vi "输入数据解析.vi"(0 "单个参数补充":dbl, 1 "从板号":dbl=1.0, 2 "主板二维码":string="BNET01", 3 "从板二维码":string="BNET01", 5 "主板引用":refnum<vi>, 7 "从板引用":refnum<vi>, 9 "主板选项":string="三级故障阀值", 11 "枚举":enum16{"主板", "从板"}(ring), 12 "快换":bool caption="快换写入") -> (4 "输出数组":dbl[][](array[numeric]), 6 "数组长度":dbl[](array[numeric]), 8 "循环次数":i32, 10 "命令":u32, 14 "名称":string[](array[string]), 15 "命令序号":u32[](array[numeric]))   [LabVIEW 2013] (continued)
                  frame Enabled {
                  }
                }
                n1001 = Build Array(w2456) -> (w2455:i32[])
              }
              frame 5 {
                # "单组电压不均衡"
                n1002 = disable-structure shown="启用" {
                  disable-tunnel: [w2472 w2475] -> w2467
                  disable-tunnel: [w2470 w2475] -> w2465
                  disable-tunnel: w2464 -> [w2469 _]
                  frame Disabled {
                    n1003 = Unbundle By Name(w2469) -> ("单组电压不均衡"=w2468:dbl)
                    n1004 = call "输入分辨率计算-EV05.vi"("1字节?"=FALSE, "数值"=w2468, "偏移量"=0.0, "分辨率"=0.001) -> ("低字节"=w2470:dbl, "高字节1"=w2472:dbl)  [unwired: 1 in, 5 out]
                  }
                  frame Enabled {
                    w2475 = 255 ("高字节1")
                  }
                }
                n1005 = Build Array(w2467, w2465) -> (w2466:i32[])
              }
              frame 6 {
                # "整组电压不均衡"
                n1006 = disable-structure shown="启用" {
                  disable-tunnel: [w2484 w2487] -> w2479
                  disable-tunnel: [w2482 w2487] -> w2477
                  disable-tunnel: w2476 -> [w2481 _]
                  frame Disabled {
                    n1007 = Unbundle By Name(w2481) -> ("整组电压不均衡"=w2480:dbl)
                    n1008 = call "输入分辨率计算-EV05.vi"("1字节?"=FALSE, "数值"=w2480, "偏移量"=0.0, "分辨率"=0.001) -> ("低字节"=w2482:dbl, "高字节1"=w2484:dbl)  [unwired: 1 in, 5 out]
                  }
                  frame Enabled {
                    w2487 = 255 ("高字节1")
                  }
                }
                n1009 = Build Array(w2479, w2477) -> (w2478:i32[])
              }
              frame 7 {
                # "单体电压过高"
                n1010 = disable-structure shown="启用" {
                  disable-tunnel: [w2496 w2499] -> w2491
                  disable-tunnel: [w2494 w2499] -> w2489
                  disable-tunnel: w2488 -> [w2493 _]
                  frame Disabled {
                    n1011 = Unbundle By Name(w2493) -> ("单体电压过高"=w2492:dbl)
                    n1012 = call "输入分辨率计算-EV05.vi"("1字节?"=FALSE, "数值"=w2492, "偏移量"=0.0, "分辨率"=0.001) -> ("低字节"=w2494:dbl, "高字节1"=w2496:dbl)  [unwired: 1 in, 5 out]
                  }
                  frame Enabled {
                    w2499 = 255 ("高字节1")
                  }
                }
                n1013 = Build Array(w2491, w2489) -> (w2490:i32[])
              }
              frame 8 {
                # "单体电压过低"
                n1014 = disable-structure shown="启用" {
                  disable-tunnel: [w2508 w2511] -> w2503
                  disable-tunnel: [w2506 w2511] -> w2501
                  disable-tunnel: w2500 -> [w2505 _]
                  frame Disabled {
                    n1015 = Unbundle By Name(w2505) -> ("单体电压过低"=w2504:dbl)
                    n1016 = call "输入分辨率计算-EV05.vi"("1字节?"=FALSE, "数值"=w2504, "偏移量"=0.0, "分辨率"=0.001) -> ("低字节"=w2506:dbl, "高字节1"=w2508:dbl)  [unwired: 1 in, 5 out]
                  }
                  frame Enabled {
                    w2511 = 255 ("高字节1")
                  }
                }
                n1017 = Build Array(w2503, w2501) -> (w2502:i32[])
              }
              frame 9 {
                # "充电电流过高"
                n1018 = disable-structure shown="启用" {
                  disable-tunnel: [w2520 w2523] -> w2515
                  disable-tunnel: [w2518 w2523] -> w2513
                  disable-tunnel: w2512 -> [w2517 _]
                  frame Disabled {
                    n1019 = Unbundle By Name(w2517) -> ("充电电流过高"=w2516:dbl)
                    n1020 = call "输入分辨率计算-EV05.vi"("1字节?"=FALSE, "数值"=w2516, "偏移量"=-3000.0, "分辨率"=0.1) -> ("低字节"=w2518:dbl, "高字节1"=w2520:dbl)  [unwired: 1 in, 5 out]
                  }
                  frame Enabled {
                    w2523 = 255 ("高字节1")
                  }
                }
                n1021 = Build Array(w2515, w2513) -> (w2514:i32[])
              }
              frame 10 {
                # "放电电流过高"
                n1022 = disable-structure shown="启用" {
                  disable-tunnel: [w2532 w2535] -> w2527
                  disable-tunnel: [w2530 w2535] -> w2525
                  disable-tunnel: w2524 -> [w2529 _]
                  frame Disabled {
                    n1023 = Unbundle By Name(w2529) -> ("放电电流过高"=w2528:dbl)
                    n1024 = call "输入分辨率计算-EV05.vi"("1字节?"=FALSE, "数值"=w2528, "偏移量"=-3000.0, "分辨率"=0.1) -> ("低字节"=w2530:dbl, "高字节1"=w2532:dbl)  [unwired: 1 in, 5 out]
                  }
                  frame Enabled {
                    w2535 = 255 ("高字节1")
                  }
                }
                n1025 = Build Array(w2527, w2525) -> (w2526:i32[])
              }
              frame 11 {
                # "单组温度不均衡"
                n1026 = disable-structure shown="启用" {
                  disable-tunnel: [w2542 255 ("高字节1")] -> w2538
                  disable-tunnel: w2536 -> [w2540 _]
                  frame Disabled {
                    n1027 = Unbundle By Name(w2540) -> ("单组温度不均衡"=w2539:dbl)
                    n1028 = call "输入分辨率计算-EV05.vi"("1字节?"=TRUE, "数值"=w2539, "偏移量"=0.0, "分辨率"=1.0) -> ("高字节1"=w2542:dbl)  [unwired: 1 in, 6 out]
                  }
                  frame Enabled {
                  }
                }
                n1029 = Build Array(w2538) -> (w2537:i32[])
              }
              frame 12 {
                # "SOC过高"
                n1030 = Unbundle By Name(w2550) -> ("SOC过高"=w2549:dbl)
                n1031 = call "输入分辨率计算-EV05.vi"("1字节?"=FALSE, "数值"=w2549, "偏移量"=0.0, "分辨率"=0.1) -> ("低字节"=w2551:dbl, "高字节1"=w2552:dbl)  [unwired: 1 in, 5 out]
                n1032 = call "二进制解析-8.6.vi"("索引"=4, "数值"=w2552) -> ("低位子数组"=w2555:i32[])  [unwired: 3 out]
                n1033 = call "二进制解析-8.6.vi"("索引"=4, "数值"=w2551) -> ("低位子数组"=w2547:i32[], "高位子数组"=w2554:i32[])  [unwired: 2 out]
                n1034 = Insert Into Array(array=w2555, new element=w2554) -> (w2553:i32[])  [unwired: 1 in]
                n1035 = call "数值二进制转十进制-8.6.vi"("子数组"=w2553) -> ("十进制数值"=w2548:i32)  [unwired: 4 out]
                n1036 = disable-structure shown="启用" {
                  disable-tunnel: w2548 -> [w2563 _]
                  disable-tunnel: [w2563 255 ("高字节1")] -> w2546
                  disable-tunnel: [w2562 i32[] [] ("低位子数组 20")] -> _
                  disable-tunnel: w2547 -> [w2562 _]
                  frame Disabled {
                  }
                  frame Enabled {
                  }
                }
                n1037 = Build Array(w2546, w2546) -> (w2559:i32[])
              }
              frame 13 {
                # "SOC过低"
                n1038 = Unbundle By Name(w2572) -> ("SOC过低"=w2571:dbl)
                n1039 = call "输入分辨率计算-EV05.vi"("1字节?"=FALSE, "数值"=w2571, "偏移量"=0.0, "分辨率"=0.1) -> ("低字节"=w2569:dbl, "高字节1"=w2570:dbl)  [unwired: 1 in, 5 out]
                n1040 = call "二进制解析-8.6.vi"("索引"=4, "数值"=w2570) -> ("低位子数组"=w2567:i32[])  [unwired: 3 out]
                n1041 = disable-structure shown="启用" {
                  disable-tunnel: w2569 -> [w2579 _]
                  disable-tunnel: [w2579 255 ("高字节1")] -> w2568
                  disable-tunnel: w2567 -> [w2578 _]
                  disable-tunnel: [_ 255 ("高字节1")] -> w2566
                  frame Disabled {
                    (unwired) i32[] [] ("低位子数组 4")
                  }
                  frame Enabled {
                  }
                }
                n1042 = Build Array(w2566, w2568) -> (w2575:i32[])
              }
              frame 14 {
                # "内阻过大"
                n1043 = disable-structure shown="启用" {
                  disable-tunnel: w2584 -> [w2589 _]
                  disable-tunnel: [w2585 255 ("高字节1")] -> w2582
                  frame Disabled {
                    n1044 = Unbundle By Name(w2589) -> ("内阻过大"=w2588:dbl)
                    n1045 = call "输入分辨率计算-EV05.vi"("1字节?"=TRUE, "数值"=w2588, "分辨率"=0.1) -> ("高字节1"=w2585:dbl)  [unwired: 2 in, 6 out]
                  }
                  frame Enabled {
                  }
                }
                n1046 = Build Array(w2582) -> (w2583:i32[])
              }
              frame 15 {
                # "极柱温度过高"
                n1047 = disable-structure shown="启用" {
                  disable-tunnel: w2593 -> [w2599 _]
                  disable-tunnel: [w2595 255 ("高字节1")] -> w2591
                  frame Disabled {
                    n1048 = Unbundle By Name(w2599) -> ("极柱温度过高"=w2598:dbl)
                    n1049 = call "输入分辨率计算-EV05.vi"("1字节?"=TRUE, "数值"=w2598, "偏移量"=-40.0, "分辨率"=1.0) -> ("高字节1"=w2595:dbl)  [unwired: 1 in, 6 out]
                  }
                  frame Enabled {
                  }
                }
                n1050 = Build Array(w2591) -> (w2592:i32[])
              }
              frame 16 {
                # "SOH过低"
                n1051 = disable-structure shown="启用" {
                  disable-tunnel: [w2616 w2624] -> w2603
                  disable-tunnel: w2602 -> [w2613 _]
                  disable-tunnel: [w2605 w2624] -> w2601
                  frame Disabled {
                    n1052 = Unbundle By Name(w2613) -> ("SOH过低"=w2612:dbl)
                    n1053 = call "输入分辨率计算-EV05.vi"("1字节?"=FALSE, "数值"=w2612, "偏移量"=0.0, "分辨率"=0.1) -> ("低字节"=w2614:dbl, "高字节1"=w2615:dbl)  [unwired: 1 in, 5 out]
                    n1054 = call "二进制解析-8.6.vi"("索引"=4, "数值"=w2615) -> ("低位子数组"=w2618:i32[])  [unwired: 3 out]
                    n1055 = call "二进制解析-8.6.vi"("索引"=4, "数值"=w2614) -> ("低位子数组"=w2607:i32[], "高位子数组"=w2617:i32[])  [unwired: 2 out]
                    n1056 = call "二进制解析-8.6.vi"("索引"=4, "数值"=0) -> ("低位子数组"=w2608:i32[])  [unwired: 3 out]
                    n1057 = Insert Into Array(array=w2618, new element=w2617) -> (w2611:i32[])  [unwired: 1 in]
                    n1058 = Insert Into Array(array=w2607, new element=w2608) -> (w2606:i32[])  [unwired: 1 in]
                    n1059 = call "数值二进制转十进制-8.6.vi"("子数组"=w2611) -> ("十进制数值"=w2616:i32)  [unwired: 4 out]
                    n1060 = call "数值二进制转十进制-8.6.vi"("子数组"=w2606) -> ("十进制数值"=w2605:i32)  [unwired: 4 out]
                  }
                  frame Enabled {
                    w2624 = 255 ("高字节1")
                  }
                }
                n1061 = Build Array(w2603, w2601) -> (w2604:i32[])
              }
            }
            n1062 = Insert Into Array(array=w2408, new element=w2409) -> (w2407:dbl[])  [unwired: 1 in]
          }
          n1063 = Build Array(w2404) -> (w2403:dbl[][])
          n1064 = Build Array("三级故障阀值") -> (w2394:string[])
        }
        frame "温度过高(2)" {
          n1065 = Unbundle By Name(w2630) -> ("一级故障 2"=w2631:refnum<vi>)
          n1066 = property class="Clust (严格)"(reference=w2631) -> ("Value"=w2629:T4)  [unwired: 1 in, 2 out]
          n1067 = for {
            N: 17 -> [_]
            tunnel: w2629 -> [w2641]
            shift-right: [w2638] -> w2635
            shift-left: dbl[] [] -> [w2639]
            i -> [w2642]
            n1068 = case shown="13" w2642 {
              tunnel: w2641 -> [w2643 w2654 w2665 w2675 w2685 w2695 w2707 w2719 w2731 w2743 w2755 w2767 w2781 w2803 w2815 w2824 w2833]
              tunnel: [w2644 w2655 w2666 w2676 w2686 w2697 w2709 w2721 w2733 w2745 w2757 w2768 w2790 w2806 w2814 w2823 w2835] -> w2640
              frame 0, Default {
                # "总电压过高"
                n1069 = disable-structure shown="启用" {
                  disable-tunnel: [w2650 w2653] -> w2646
                  disable-tunnel: [w2649 w2653] -> w2645
                  disable-tunnel: w2643 -> [w2648 _]
                  frame Disabled {
                    n1070 = Unbundle By Name(w2648) -> ("总电压过高"=w2647:dbl)
                    n1071 = call "输入分辨率计算-EV05.vi"("1字节?"=FALSE, "数值"=w2647, "分辨率"=0.1) -> ("低字节"=w2650:dbl, "高字节1"=w2649:dbl)  [unwired: 2 in, 5 out]
                  }
                  frame Enabled {
                    w2653 = 255 ("高字节1")
                  }
                }
                n1072 = Build Array(w2645, w2646) -> (w2644:i32[])
              }
              frame 1 {
                # "总电压过低"
                n1073 = disable-structure shown="启用" {
                  disable-tunnel: [w2661 w2664] -> w2657
                  disable-tunnel: [w2660 w2664] -> w2656
                  disable-tunnel: w2654 -> [w2659 _]
                  frame Disabled {
                    n1074 = Unbundle By Name(w2659) -> ("总电压过低"=w2658:dbl)
                    n1075 = call "输入分辨率计算-EV05.vi"("1字节?"=FALSE, "数值"=w2658, "分辨率"=0.1) -> ("低字节"=w2661:dbl, "高字节1"=w2660:dbl)  [unwired: 2 in, 5 out]
                  }
                  frame Enabled {
                    w2664 = 255 ("高字节1")
                  }
                }
                n1076 = Build Array(w2656, w2657) -> (w2655:i32[])
              }
              frame 2 {
                # "温度过高"
                n1077 = disable-structure shown="启用" {
                  disable-tunnel: [w2671 255 ("高字节1")] -> w2667
                  disable-tunnel: w2665 -> [w2669 _]
                  frame Enabled {
                    n1078 = Unbundle By Name(w2669) -> ("温度过高"=w2668:dbl)
                    n1079 = call "输入分辨率计算-EV05.vi"("1字节?"=TRUE, "数值"=w2668, "偏移量"=-40.0, "分辨率"=1.0) -> ("高字节1"=w2671:dbl)  [unwired: 1 in, 6 out]
                  }
                  frame Disabled {
                  }
                }
                n1080 = Build Array(w2667) -> (w2666:dbl[])
              }
              frame 3 {
                # "温度过低"
                n1081 = disable-structure shown="启用" {
                  disable-tunnel: [w2681 255 ("高字节1")] -> w2677
                  disable-tunnel: w2675 -> [w2679 _]
                  frame Disabled {
                    n1082 = Unbundle By Name(w2679) -> ("温度过低"=w2678:dbl)
                    n1083 = call "输入分辨率计算-EV05.vi"("1字节?"=TRUE, "数值"=w2678, "偏移量"=-40.0, "分辨率"=1.0) -> ("高字节1"=w2681:dbl)  [unwired: 1 in, 6 out]
                  }
                  frame Enabled {
                  }
                }
                n1084 = Build Array(w2677) -> (w2676:i32[])
              }
              frame 4 {
                # "整组温度不均衡"
                n1085 = disable-structure shown="启用" {
                  disable-tunnel: [w2691 255 ("高字节1")] -> w2687
                  disable-tunnel: w2685 -> [w2689 _]
                  frame Disabled {
                    n1086 = Unbundle By Name(w2689) -> ("整组温度不均衡"=w2688:dbl)
                    n1087 = call "输入分辨率计算-EV05.vi"("1字节?"=TRUE, "数值"=w2688, "偏移量"=0.0, "分辨率"=1.0) -> ("高字节1"=w2691:dbl)  [unwired: 1 in, 6 out]
                  }
                  frame Enabled {
                  }
                }
                n1088 = Build Array(w2687) -> (w2686:i32[])
              }
              frame 5 {
                # "单组电压不均衡"
                n1089 = disable-structure shown="启用" {
                  disable-tunnel: [w2703 w2706] -> w2698
                  disable-tunnel: [w2701 w2706] -> w2696
                  disable-tunnel: w2695 -> [w2700 _]
                  frame Disabled {
                    n1090 = Unbundle By Name(w2700) -> ("单组电压不均衡"=w2699:dbl)
                    n1091 = call "输入分辨率计算-EV05.vi"("1字节?"=FALSE, "数值"=w2699, "偏移量"=0.0, "分辨率"=0.001) -> ("低字节"=w2701:dbl, "高字节1"=w2703:dbl)  [unwired: 1 in, 5 out]
                  }
                  frame Enabled {
                    w2706 = 255 ("高字节1")
                  }
                }
                n1092 = Build Array(w2698, w2696) -> (w2697:i32[])
              }
              frame 6 {
                # "整组电压不均衡"
                n1093 = disable-structure shown="启用" {
                  disable-tunnel: [w2715 w2718] -> w2710
                  disable-tunnel: [w2713 w2718] -> w2708
                  disable-tunnel: w2707 -> [w2712 _]
                  frame Disabled {
                    n1094 = Unbundle By Name(w2712) -> ("整组电压不均衡"=w2711:dbl)
                    n1095 = call "输入分辨率计算-EV05.vi"("1字节?"=FALSE, "数值"=w2711, "偏移量"=0.0, "分辨率"=0.001) -> ("低字节"=w2713:dbl, "高字节1"=w2715:dbl)  [unwired: 1 in, 5 out]
                  }
                  frame Enabled {
                    w2718 = 255 ("高字节1")
                  }
                }
                n1096 = Build Array(w2710, w2708) -> (w2709:i32[])
              }
              frame 7 {
                # "单体电压过高"
                n1097 = disable-structure shown="启用" {
                  disable-tunnel: [w2727 w2730] -> w2722
                  disable-tunnel: [w2725 w2730] -> w2720
                  disable-tunnel: w2719 -> [w2724 _]
                  frame Disabled {
                    n1098 = Unbundle By Name(w2724) -> ("单体电压过高"=w2723:dbl)
                    n1099 = call "输入分辨率计算-EV05.vi"("1字节?"=FALSE, "数值"=w2723, "偏移量"=0.0, "分辨率"=0.001) -> ("低字节"=w2725:dbl, "高字节1"=w2727:dbl)  [unwired: 1 in, 5 out]
                  }
                  frame Enabled {
                    w2730 = 255 ("高字节1")
                  }
                }
                n1100 = Build Array(w2722, w2720) -> (w2721:i32[])
              }
              frame 8 {
                # "单体电压过低"
                n1101 = disable-structure shown="启用" {
                  disable-tunnel: [w2739 w2742] -> w2734
                  disable-tunnel: [w2737 w2742] -> w2732
                  disable-tunnel: w2731 -> [w2736 _]
                  frame Disabled {
                    n1102 = Unbundle By Name(w2736) -> ("单体电压过低"=w2735:dbl)
                    n1103 = call "输入分辨率计算-EV05.vi"("1字节?"=FALSE, "数值"=w2735, "偏移量"=0.0, "分辨率"=0.001) -> ("低字节"=w2737:dbl, "高字节1"=w2739:dbl)  [unwired: 1 in, 5 out]
                  }
                  frame Enabled {
                    w2742 = 255 ("高字节1")
                  }
                }
                n1104 = Build Array(w2734, w2732) -> (w2733:i32[])
              }
              frame 9 {
                # "充电电流过高"
                n1105 = disable-structure shown="启用" {
                  disable-tunnel: [w2751 w2754] -> w2746
                  disable-tunnel: [w2749 w2754] -> w2744
                  disable-tunnel: w2743 -> [w2748 _]
                  frame Disabled {
                    n1106 = Unbundle By Name(w2748) -> ("充电电流过高"=w2747:dbl)
                    n1107 = call "输入分辨率计算-EV05.vi"("1字节?"=FALSE, "数值"=w2747, "偏移量"=-3000.0, "分辨率"=0.1) -> ("低字节"=w2749:dbl, "高字节1"=w2751:dbl)  [unwired: 1 in, 5 out]
                  }
                  frame Enabled {
                    w2754 = 255 ("高字节1")
                  }
                }
                n1108 = Build Array(w2746, w2744) -> (w2745:i32[])
              }
              frame 10 {
                # "放电电流过高"
                n1109 = disable-structure shown="启用" {
                  disable-tunnel: [w2763 w2766] -> w2758
                  disable-tunnel: [w2761 w2766] -> w2756
                  disable-tunnel: w2755 -> [w2760 _]
                  frame Disabled {
                    n1110 = Unbundle By Name(w2760) -> ("放电电流过高"=w2759:dbl)
                    n1111 = call "输入分辨率计算-EV05.vi"("1字节?"=FALSE, "数值"=w2759, "偏移量"=-3000.0, "分辨率"=0.1) -> ("低字节"=w2761:dbl, "高字节1"=w2763:dbl)  [unwired: 1 in, 5 out]
                  }
                  frame Enabled {
                    w2766 = 255 ("高字节1")
                  }
                }
                n1112 = Build Array(w2758, w2756) -> (w2757:i32[])
              }
              frame 11 {
                # "单组温度不均衡"
                n1113 = disable-structure shown="启用" {
                  disable-tunnel: [w2773 255 ("高字节1")] -> w2769
                  disable-tunnel: w2767 -> [w2771 _]
                  frame Disabled {
                    n1114 = Unbundle By Name(w2771) -> ("单组温度不均衡"=w2770:dbl)
                    n1115 = call "输入分辨率计算-EV05.vi"("1字节?"=TRUE, "数值"=w2770, "偏移量"=0.0, "分辨率"=1.0) -> ("高字节1"=w2773:dbl)  [unwired: 1 in, 6 out]
                  }
                  frame Enabled {
                  }
                }
                n1116 = Build Array(w2769) -> (w2768:i32[])
              }
              frame 12 {
                # "SOC过高"
                n1117 = Unbundle By Name(w2781) -> ("SOC过高"=w2780:dbl)
                n1118 = call "输入分辨率计算-EV05.vi"("1字节?"=FALSE, "数值"=w2780, "偏移量"=0.0, "分辨率"=0.1) -> ("低字节"=w2782:dbl, "高字节1"=w2783:dbl)  [unwired: 1 in, 5 out]
                n1119 = call "二进制解析-8.6.vi"("索引"=4, "数值"=w2783) -> ("低位子数组"=w2786:i32[])  [unwired: 3 out]
                n1120 = call "二进制解析-8.6.vi"("索引"=4, "数值"=w2782) -> ("低位子数组"=w2778:i32[], "高位子数组"=w2785:i32[])  [unwired: 2 out]
                n1121 = Insert Into Array(array=w2786, new element=w2785) -> (w2784:i32[])  [unwired: 1 in]
                n1122 = call "数值二进制转十进制-8.6.vi"("子数组"=w2784) -> ("十进制数值"=w2779:i32)  [unwired: 4 out]
                n1123 = disable-structure shown="启用" {
                  disable-tunnel: w2779 -> [w2794 _]
                  disable-tunnel: [w2794 255 ("高字节1")] -> w2777
                  disable-tunnel: [w2793 i32[] [] ("低位子数组 20")] -> _
                  disable-tunnel: w2778 -> [w2793 _]
                  frame Disabled {
                  }
                  frame Enabled {
                  }
                }
                n1124 = Build Array(w2777, w2777) -> (w2790:i32[])
              }
              frame 13 {
                # "SOC过低"
                n1125 = Unbundle By Name(w2803) -> ("SOC过低"=w2802:dbl)
                n1126 = call "输入分辨率计算-EV05.vi"("1字节?"=FALSE, "数值"=w2802, "偏移量"=0.0, "分辨率"=0.1) -> ("低字节"=w2800:dbl, "高字节1"=w2801:dbl)  [unwired: 1 in, 5 out]
                n1127 = call "二进制解析-8.6.vi"("索引"=4, "数值"=w2801) -> ("低位子数组"=w2798:i32[])  [unwired: 3 out]
                n1128 = disable-structure shown="启用" {
                  disable-tunnel: w2800 -> [w2810 _]
                  disable-tunnel: [w2810 255 ("高字节1")] -> w2799
                  disable-tunnel: w2798 -> [w2809 _]
                  disable-tunnel: [_ 255 ("高字节1")] -> w2797
                  frame Disabled {
                    (unwired) i32[] [] ("低位子数组 4")
                  }
                  frame Enabled {
                  }
                }
                n1129 = Build Array(w2797, w2799) -> (w2806:i32[])
              }
              frame 14 {
                # "内阻过大"
                n1130 = disable-structure shown="启用" {
                  disable-tunnel: w2815 -> [w2820 _]
                  disable-tunnel: [w2816 255 ("高字节1")] -> w2813
                  frame Disabled {
                    n1131 = Unbundle By Name(w2820) -> ("内阻过大"=w2819:dbl)
                    n1132 = call "输入分辨率计算-EV05.vi"("1字节?"=TRUE, "数值"=w2819, "分辨率"=0.1) -> ("高字节1"=w2816:dbl)  [unwired: 2 in, 6 out]
                  }
                  frame Enabled {
                  }
                }
                n1133 = Build Array(w2813) -> (w2814:i32[])
              }
              frame 15 {
                # "极柱温度过高"
                n1134 = disable-structure shown="启用" {
                  disable-tunnel: w2824 -> [w2830 _]
                  disable-tunnel: [w2826 255 ("高字节1")] -> w2822
                  frame Disabled {
                    n1135 = Unbundle By Name(w2830) -> ("极柱温度过高"=w2829:dbl)
                    n1136 = call "输入分辨率计算-EV05.vi"("1字节?"=TRUE, "数值"=w2829, "偏移量"=-40.0, "分辨率"=1.0) -> ("高字节1"=w2826:dbl)  [unwired: 1 in, 6 out]
                  }
                  frame Enabled {
                  }
                }
                n1137 = Build Array(w2822) -> (w2823:i32[])
              }
              frame 16 {
                # "SOH过低"
                n1138 = disable-structure shown="启用" {
                  disable-tunnel: [w2847 w2855] -> w2834
                  disable-tunnel: w2833 -> [w2844 _]
                  disable-tunnel: [w2836 w2855] -> w2832
                  frame Disabled {
                    n1139 = Unbundle By Name(w2844) -> ("SOH过低"=w2843:dbl)
                    n1140 = call "输入分辨率计算-EV05.vi"("1字节?"=FALSE, "数值"=w2843, "偏移量"=0.0, "分辨率"=0.1) -> ("低字节"=w2845:dbl, "高字节1"=w2846:dbl)  [unwired: 1 in, 5 out]
                    n1141 = call "二进制解析-8.6.vi"("索引"=4, "数值"=w2846) -> ("低位子数组"=w2849:i32[])  [unwired: 3 out]
                    n1142 = call "二进制解析-8.6.vi"("索引"=4, "数值"=w2845) -> ("低位子数组"=w2838:i32[], "高位子数组"=w2848:i32[])  [unwired: 2 out]
                    n1143 = call "二进制解析-8.6.vi"("索引"=4, "数值"=0) -> ("低位子数组"=w2839:i32[])  [unwired: 3 out]
                    n1144 = Insert Into Array(array=w2849, new element=w2848) -> (w2842:i32[])  [unwired: 1 in]
                    n1145 = Insert Into Array(array=w2838, new element=w2839) -> (w2837:i32[])  [unwired: 1 in]
                    n1146 = call "数值二进制转十进制-8.6.vi"("子数组"=w2842) -> ("十进制数值"=w2847:i32)  [unwired: 4 out]
                    n1147 = call "数值二进制转十进制-8.6.vi"("子数组"=w2837) -> ("十进制数值"=w2836:i32)  [unwired: 4 out]
                  }
                  frame Enabled {
                    w2855 = 255 ("高字节1")
                  }
                }
                n1148 = Build Array(w2834, w2832) -> (w2835:i32[])
              }
            }
            n1149 = Insert Into Array(array=w2639, new element=w2640) -> (w2638:dbl[])  [unwired: 1 in]
          }
          n1150 = Build Array(w2635) -> (w2634:dbl[][])
          n1151 = Build Array("二级故障阀值") -> (w2625:string[])
        }
        frame "温度过高(3)" {
          n1152 = Unbundle By Name(w2861) -> ("一级故障 3"=w2862:refnum<vi>)
          n1153 = property class="Clust (严格)"(reference=w2862) -> ("Value"=w2860:T4)  [unwired: 1 in, 2 out]
          n1154 = for {
            N: 17 -> [_]
            tunnel: w2860 -> [w2872]
            shift-right: [w2869] -> w2866
            shift-left: dbl[] [] -> [w2870]
            i -> [w2873]
            n1155 = case shown="13" w2873 {
              tunnel: w2872 -> [w2874 w2885 w2896 w2906 w2916 w2926 w2938 w2950 w2962 w2974 w2986 w2998 w3012 w3034 w3046 w3055 w3064]
              tunnel: [w2875 w2886 w2897 w2907 w2917 w2928 w2940 w2952 w2964 w2976 w2988 w2999 w3021 w3037 w3045 w3054 w3066] -> w2871
              frame 0, Default {
                # "总电压过高"
                n1156 = disable-structure shown="启用" {
                  disable-tunnel: [w2881 w2884] -> w2877
                  disable-tunnel: [w2880 w2884] -> w2876
                  disable-tunnel: w2874 -> [w2879 _]
                  frame Disabled {
                    n1157 = Unbundle By Name(w2879) -> ("总电压过高"=w2878:dbl)
                    n1158 = call "输入分辨率计算-EV05.vi"("1字节?"=FALSE, "数值"=w2878, "分辨率"=0.1) -> ("低字节"=w2881:dbl, "高字节1"=w2880:dbl)  [unwired: 2 in, 5 out]
                  }
                  frame Enabled {
                    w2884 = 255 ("高字节1")
                  }
                }
                n1159 = Build Array(w2876, w2877) -> (w2875:i32[])
              }
              frame 1 {
                # "总电压过低"
                n1160 = disable-structure shown="启用" {
                  disable-tunnel: [w2892 w2895] -> w2888
                  disable-tunnel: [w2891 w2895] -> w2887
                  disable-tunnel: w2885 -> [w2890 _]
                  frame Disabled {
                    n1161 = Unbundle By Name(w2890) -> ("总电压过低"=w2889:dbl)
                    n1162 = call "输入分辨率计算-EV05.vi"("1字节?"=FALSE, "数值"=w2889, "分辨率"=0.1) -> ("低字节"=w2892:dbl, "高字节1"=w2891:dbl)  [unwired: 2 in, 5 out]
                  }
                  frame Enabled {
                    w2895 = 255 ("高字节1")
                  }
                }
                n1163 = Build Array(w2887, w2888) -> (w2886:i32[])
              }
              frame 2 {
                # "温度过高"
                n1164 = disable-structure shown="启用" {
                  disable-tunnel: [w2902 255 ("高字节1")] -> w2898
                  disable-tunnel: w2896 -> [w2900 _]
                  frame Enabled {
                    n1165 = Unbundle By Name(w2900) -> ("温度过高"=w2899:dbl)
                    n1166 = call "输入分辨率计算-EV05.vi"("1字节?"=TRUE, "数值"=w2899, "偏移量"=-40.0, "分辨率"=1.0) -> ("高字节1"=w2902:dbl)  [unwired: 1 in, 6 out]
                  }
                  frame Disabled {
                  }
                }
                n1167 = Build Array(w2898) -> (w2897:dbl[])
              }
              frame 3 {
                # "温度过低"
                n1168 = disable-structure shown="启用" {
                  disable-tunnel: [w2912 255 ("高字节1")] -> w2908
                  disable-tunnel: w2906 -> [w2910 _]
                  frame Disabled {
                    n1169 = Unbundle By Name(w2910) -> ("温度过低"=w2909:dbl)
                    n1170 = call "输入分辨率计算-EV05.vi"("1字节?"=TRUE, "数值"=w2909, "偏移量"=-40.0, "分辨率"=1.0) -> ("高字节1"=w2912:dbl)  [unwired: 1 in, 6 out]
                  }
                  frame Enabled {
                  }
                }
                n1171 = Build Array(w2908) -> (w2907:i32[])
              }
              frame 4 {
                # "整组温度不均衡"
                n1172 = disable-structure shown="启用" {
                  disable-tunnel: [w2922 255 ("高字节1")] -> w2918
                  disable-tunnel: w2916 -> [w2920 _]
                  frame Disabled {
                    n1173 = Unbundle By Name(w2920) -> ("整组温度不均衡"=w2919:dbl)
                    n1174 = call "输入分辨率计算-EV05.vi"("1字节?"=TRUE, "数值"=w2919, "偏移量"=0.0, "分辨率"=1.0) -> ("高字节1"=w2922:dbl)  [unwired: 1 in, 6 out]
                  }
                  frame Enabled {
                  }
                }
                n1175 = Build Array(w2918) -> (w2917:i32[])
              }
              frame 5 {
                # "单组电压不均衡"
                n1176 = disable-structure shown="启用" {
                  disable-tunnel: [w2934 w2937] -> w2929
                  disable-tunnel: [w2932 w2937] -> w2927
                  disable-tunnel: w2926 -> [w2931 _]
                  frame Disabled {
                    n1177 = Unbundle By Name(w2931) -> ("单组电压不均衡"=w2930:dbl)
                    n1178 = call "输入分辨率计算-EV05.vi"("1字节?"=FALSE, "数值"=w2930, "偏移量"=0.0, "分辨率"=0.001) -> ("低字节"=w2932:dbl, "高字节1"=w2934:dbl)  [unwired: 1 in, 5 out]
                  }
                  frame Enabled {
                    w2937 = 255 ("高字节1")
                  }
                }
                n1179 = Build Array(w2929, w2927) -> (w2928:i32[])
              }
              frame 6 {
                # "整组电压不均衡"
                n1180 = disable-structure shown="启用" {
                  disable-tunnel: [w2946 w2949] -> w2941
                  disable-tunnel: [w2944 w2949] -> w2939
                  disable-tunnel: w2938 -> [w2943 _]
                  frame Disabled {
                    n1181 = Unbundle By Name(w2943) -> ("整组电压不均衡"=w2942:dbl)
                    n1182 = call "输入分辨率计算-EV05.vi"("1字节?"=FALSE, "数值"=w2942, "偏移量"=0.0, "分辨率"=0.001) -> ("低字节"=w2944:dbl, "高字节1"=w2946:dbl)  [unwired: 1 in, 5 out]
                  }
                  frame Enabled {
                    w2949 = 255 ("高字节1")
                  }
                }
                n1183 = Build Array(w2941, w2939) -> (w2940:i32[])
              }
              frame 7 {
                # "单体电压过高"
                n1184 = disable-structure shown="启用" {
                  disable-tunnel: [w2958 w2961] -> w2953
                  disable-tunnel: [w2956 w2961] -> w2951
                  disable-tunnel: w2950 -> [w2955 _]
                  frame Disabled {
                    n1185 = Unbundle By Name(w2955) -> ("单体电压过高"=w2954:dbl)
                    n1186 = call "输入分辨率计算-EV05.vi"("1字节?"=FALSE, "数值"=w2954, "偏移量"=0.0, "分辨率"=0.001) -> ("低字节"=w2956:dbl, "高字节1"=w2958:dbl)  [unwired: 1 in, 5 out]
                  }
                  frame Enabled {
                    w2961 = 255 ("高字节1")
                  }
                }
                n1187 = Build Array(w2953, w2951) -> (w2952:i32[])
              }
              frame 8 {
                # "单体电压过低"
                n1188 = disable-structure shown="启用" {
                  disable-tunnel: [w2970 w2973] -> w2965
                  disable-tunnel: [w2968 w2973] -> w2963
                  disable-tunnel: w2962 -> [w2967 _]
                  frame Disabled {
                    n1189 = Unbundle By Name(w2967) -> ("单体电压过低"=w2966:dbl)
                    n1190 = call "输入分辨率计算-EV05.vi"("1字节?"=FALSE, "数值"=w2966, "偏移量"=0.0, "分辨率"=0.001) -> ("低字节"=w2968:dbl, "高字节1"=w2970:dbl)  [unwired: 1 in, 5 out]
                  }
                  frame Enabled {
                    w2973 = 255 ("高字节1")
                  }
                }
                n1191 = Build Array(w2965, w2963) -> (w2964:i32[])
              }
              frame 9 {
                # "充电电流过高"
                n1192 = disable-structure shown="启用" {
                  disable-tunnel: [w2982 w2985] -> w2977
                  disable-tunnel: [w2980 w2985] -> w2975
                  disable-tunnel: w2974 -> [w2979 _]
                  frame Disabled {
                    n1193 = Unbundle By Name(w2979) -> ("充电电流过高"=w2978:dbl)
                    n1194 = call "输入分辨率计算-EV05.vi"("1字节?"=FALSE, "数值"=w2978, "偏移量"=-3000.0, "分辨率"=0.1) -> ("低字节"=w2980:dbl, "高字节1"=w2982:dbl)  [unwired: 1 in, 5 out]
                  }
                  frame Enabled {
                    w2985 = 255 ("高字节1")
                  }
                }
                n1195 = Build Array(w2977, w2975) -> (w2976:i32[])
              }
              frame 10 {
                # "放电电流过高"
                n1196 = disable-structure shown="启用" {
                  disable-tunnel: [w2994 w2997] -> w2989
                  disable-tunnel: [w2992 w2997] -> w2987
                  disable-tunnel: w2986 -> [w2991 _]
                  frame Disabled {
                    n1197 = Unbundle By Name(w2991) -> ("放电电流过高"=w2990:dbl)
                    n1198 = call "输入分辨率计算-EV05.vi"("1字节?"=FALSE, "数值"=w2990, "偏移量"=-3000.0, "分辨率"=0.1) -> ("低字节"=w2992:dbl, "高字节1"=w2994:dbl)  [unwired: 1 in, 5 out]
                  }
                  frame Enabled {
                    w2997 = 255 ("高字节1")
                  }
                }
                n1199 = Build Array(w2989, w2987) -> (w2988:i32[])
              }
              frame 11 {
                # "单组温度不均衡"
                n1200 = disable-structure shown="启用" {
                  disable-tunnel: [w3004 255 ("高字节1")] -> w3000
                  disable-tunnel: w2998 -> [w3002 _]
                  frame Disabled {
                    n1201 = Unbundle By Name(w3002) -> ("单组温度不均衡"=w3001:dbl)
                    n1202 = call "输入分辨率计算-EV05.vi"("1字节?"=TRUE, "数值"=w3001, "偏移量"=0.0, "分辨率"=1.0) -> ("高字节1"=w3004:dbl)  [unwired: 1 in, 6 out]
                  }
                  frame Enabled {
                  }
                }
                n1203 = Build Array(w3000) -> (w2999:i32[])
              }
              frame 12 {
                # "SOC过高"
                n1204 = Unbundle By Name(w3012) -> ("SOC过高"=w3011:dbl)
                n1205 = call "输入分辨率计算-EV05.vi"("1字节?"=FALSE, "数值"=w3011, "偏移量"=0.0, "分辨率"=0.1) -> ("低字节"=w3013:dbl, "高字节1"=w3014:dbl)  [unwired: 1 in, 5 out]
                n1206 = call "二进制解析-8.6.vi"("索引"=4, "数值"=w3014) -> ("低位子数组"=w3017:i32[])  [unwired: 3 out]
                n1207 = call "二进制解析-8.6.vi"("索引"=4, "数值"=w3013) -> ("低位子数组"=w3009:i32[], "高位子数组"=w3016:i32[])  [unwired: 2 out]
                n1208 = Insert Into Array(array=w3017, new element=w3016) -> (w3015:i32[])  [unwired: 1 in]
                n1209 = call "数值二进制转十进制-8.6.vi"("子数组"=w3015) -> ("十进制数值"=w3010:i32)  [unwired: 4 out]
                n1210 = disable-structure shown="启用" {
                  disable-tunnel: w3010 -> [w3025 _]
                  disable-tunnel: [w3025 255 ("高字节1")] -> w3008
                  disable-tunnel: [w3024 i32[] [] ("低位子数组 20")] -> _
                  disable-tunnel: w3009 -> [w3024 _]
                  frame Disabled {
                  }
                  frame Enabled {
                  }
                }
                n1211 = Build Array(w3008, w3008) -> (w3021:i32[])
              }
              frame 13 {
                # "SOC过低"
                n1212 = Unbundle By Name(w3034) -> ("SOC过低"=w3033:dbl)
                n1213 = call "输入分辨率计算-EV05.vi"("1字节?"=FALSE, "数值"=w3033, "偏移量"=0.0, "分辨率"=0.1) -> ("低字节"=w3031:dbl, "高字节1"=w3032:dbl)  [unwired: 1 in, 5 out]
                n1214 = call "二进制解析-8.6.vi"("索引"=4, "数值"=w3032) -> ("低位子数组"=w3029:i32[])  [unwired: 3 out]
                n1215 = disable-structure shown="启用" {
                  disable-tunnel: w3031 -> [w3041 _]
                  disable-tunnel: [w3041 255 ("高字节1")] -> w3030
                  disable-tunnel: w3029 -> [w3040 _]
                  disable-tunnel: [_ 255 ("高字节1")] -> w3028
                  frame Disabled {
                    (unwired) i32[] [] ("低位子数组 4")
                  }
                  frame Enabled {
                  }
                }
                n1216 = Build Array(w3028, w3030) -> (w3037:i32[])
              }
              frame 14 {
                # "内阻过大"
                n1217 = disable-structure shown="启用" {
                  disable-tunnel: w3046 -> [w3051 _]
                  disable-tunnel: [w3047 255 ("高字节1")] -> w3044
                  frame Disabled {
                    n1218 = Unbundle By Name(w3051) -> ("内阻过大"=w3050:dbl)
                    n1219 = call "输入分辨率计算-EV05.vi"("1字节?"=TRUE, "数值"=w3050, "分辨率"=0.1) -> ("高字节1"=w3047:dbl)  [unwired: 2 in, 6 out]
                  }
                  frame Enabled {
                  }
                }
                n1220 = Build Array(w3044) -> (w3045:i32[])
              }
              frame 15 {
                # "极柱温度过高"
                n1221 = disable-structure shown="启用" {
                  disable-tunnel: w3055 -> [w3061 _]
                  disable-tunnel: [w3057 255 ("高字节1")] -> w3053
                  frame Disabled {
                    n1222 = Unbundle By Name(w3061) -> ("极柱温度过高"=w3060:dbl)
                    n1223 = call "输入分辨率计算-EV05.vi"("1字节?"=TRUE, "数值"=w3060, "偏移量"=-40.0, "分辨率"=1.0) -> ("高字节1"=w3057:dbl)  [unwired: 1 in, 6 out]
                  }
                  frame Enabled {
                  }
                }
                n1224 = Build Array(w3053) -> (w3054:i32[])
              }
              frame 16 {
                # "SOH过低"
                n1225 = disable-structure shown="启用" {
                  disable-tunnel: [w3078 w3086] -> w3065
                  disable-tunnel: w3064 -> [w3075 _]
                  disable-tunnel: [w3067 w3086] -> w3063
                  frame Disabled {
                    n1226 = Unbundle By Name(w3075) -> ("SOH过低"=w3074:dbl)
                    n1227 = call "输入分辨率计算-EV05.vi"("1字节?"=FALSE, "数值"=w3074, "偏移量"=0.0, "分辨率"=0.1) -> ("低字节"=w3076:dbl, "高字节1"=w3077:dbl)  [unwired: 1 in, 5 out]
                    n1228 = call "二进制解析-8.6.vi"("索引"=4, "数值"=w3077) -> ("低位子数组"=w3080:i32[])  [unwired: 3 out]
                    n1229 = call "二进制解析-8.6.vi"("索引"=4, "数值"=w3076) -> ("低位子数组"=w3069:i32[], "高位子数组"=w3079:i32[])  [unwired: 2 out]
                    n1230 = call "二进制解析-8.6.vi"("索引"=4, "数值"=0) -> ("低位子数组"=w3070:i32[])  [unwired: 3 out]
                    n1231 = Insert Into Array(array=w3080, new element=w3079) -> (w3073:i32[])  [unwired: 1 in]
                    n1232 = Insert Into Array(array=w3069, new element=w3070) -> (w3068:i32[])  [unwired: 1 in]
                    n1233 = call "数值二进制转十进制-8.6.vi"("子数组"=w3073) -> ("十进制数值"=w3078:i32)  [unwired: 4 out]
                    n1234 = call "数值二进制转十进制-8.6.vi"("子数组"=w3068) -> ("十进制数值"=w3067:i32)  [unwired: 4 out]
                  }
                  frame Enabled {
                    w3086 = 255 ("高字节1")
                  }
                }
                n1235 = Build Array(w3065, w3063) -> (w3066:i32[])
              }
            }
            n1236 = Insert Into Array(array=w2870, new element=w2871) -> (w2869:dbl[])  [unwired: 1 in]
          }
          n1237 = Build Array(w2866) -> (w2865:dbl[][])
          n1238 = Build Array("三级故障阀值") -> (w2856:string[])
        }
        frame "温度过低" {
          n1239 = Unbundle By Name(w3092) -> ("一级故障"=w3093:refnum<vi>)
          n1240 = property class="Clust (严格)"(reference=w3093) -> ("Value"=w3091:T4)  [unwired: 1 in, 2 out]
          n1241 = for {
            N: 17 -> [_]
            tunnel: w3091 -> [w3103]
            shift-right: [w3100] -> w3097
            shift-left: dbl[] [] -> [w3101]
            i -> [w3104]
            n1242 = case shown="13" w3104 {
              tunnel: w3103 -> [w3105 w3116 w3127 w3137 w3147 w3157 w3169 w3181 w3193 w3205 w3217 w3229 w3243 w3265 w3277 w3286 w3295]
              tunnel: [w3106 w3117 w3128 w3138 w3148 w3159 w3171 w3183 w3195 w3207 w3219 w3230 w3252 w3268 w3276 w3285 w3297] -> w3102
              frame 0, Default {
                # "总电压过高"
                n1243 = disable-structure shown="启用" {
                  disable-tunnel: [w3112 w3115] -> w3108
                  disable-tunnel: [w3111 w3115] -> w3107
                  disable-tunnel: w3105 -> [w3110 _]
                  frame Disabled {
                    n1244 = Unbundle By Name(w3110) -> ("总电压过高"=w3109:dbl)
                    n1245 = call "输入分辨率计算-EV05.vi"("1字节?"=FALSE, "数值"=w3109, "分辨率"=0.1) -> ("低字节"=w3112:dbl, "高字节1"=w3111:dbl)  [unwired: 2 in, 5 out]
                  }
                  frame Enabled {
                    w3115 = 255 ("高字节1")
                  }
                }
                n1246 = Build Array(w3107, w3108) -> (w3106:i32[])
              }
              frame 1 {
                # "总电压过低"
                n1247 = disable-structure shown="启用" {
                  disable-tunnel: [w3123 w3126] -> w3119
                  disable-tunnel: [w3122 w3126] -> w3118
                  disable-tunnel: w3116 -> [w3121 _]
                  frame Disabled {
                    n1248 = Unbundle By Name(w3121) -> ("总电压过低"=w3120:dbl)
                    n1249 = call "输入分辨率计算-EV05.vi"("1字节?"=FALSE, "数值"=w3120, "分辨率"=0.1) -> ("低字节"=w3123:dbl, "高字节1"=w3122:dbl)  [unwired: 2 in, 5 out]
                  }
                  frame Enabled {
                    w3126 = 255 ("高字节1")
                  }
                }
                n1250 = Build Array(w3118, w3119) -> (w3117:i32[])
              }
              frame 2 {
                # "温度过高"
                n1251 = disable-structure shown="启用" {
                  disable-tunnel: [w3133 255 ("高字节1")] -> w3129
                  disable-tunnel: w3127 -> [w3131 _]
                  frame Disabled {
                    n1252 = Unbundle By Name(w3131) -> ("温度过高"=w3130:dbl)
                    n1253 = call "输入分辨率计算-EV05.vi"("1字节?"=TRUE, "数值"=w3130, "偏移量"=-40.0, "分辨率"=1.0) -> ("高字节1"=w3133:dbl)  [unwired: 1 in, 6 out]
                  }
                  frame Enabled {
                  }
                }
                n1254 = Build Array(w3129) -> (w3128:i32[])
              }
              frame 3 {
                # "温度过低"
                n1255 = disable-structure shown="启用" {
                  disable-tunnel: [w3143 255 ("高字节1")] -> w3139
                  disable-tunnel: w3137 -> [w3141 _]
                  frame Enabled {
                    n1256 = Unbundle By Name(w3141) -> ("温度过低"=w3140:dbl)
                    n1257 = call "输入分辨率计算-EV05.vi"("1字节?"=TRUE, "数值"=w3140, "偏移量"=-40.0, "分辨率"=1.0) -> ("高字节1"=w3143:dbl)  [unwired: 1 in, 6 out]
                  }
                  frame Disabled {
                  }
                }
                n1258 = Build Array(w3139) -> (w3138:dbl[])
              }
              frame 4 {
                # "整组温度不均衡"
                n1259 = disable-structure shown="启用" {
                  disable-tunnel: [w3153 255 ("高字节1")] -> w3149
                  disable-tunnel: w3147 -> [w3151 _]
                  frame Disabled {
                    n1260 = Unbundle By Name(w3151) -> ("整组温度不均衡"=w3150:dbl)
                    n1261 = call "输入分辨率计算-EV05.vi"("1字节?"=TRUE, "数值"=w3150, "偏移量"=0.0, "分辨率"=1.0) -> ("高字节1"=w3153:dbl)  [unwired: 1 in, 6 out]
                  }
                  frame Enabled {
                  }
                }
                n1262 = Build Array(w3149) -> (w3148:i32[])
              }
              frame 5 {
                # "单组电压不均衡"
                n1263 = disable-structure shown="启用" {
                  disable-tunnel: [w3165 w3168] -> w3160
                  disable-tunnel: [w3163 w3168] -> w3158
                  disable-tunnel: w3157 -> [w3162 _]
                  frame Disabled {
                    n1264 = Unbundle By Name(w3162) -> ("单组电压不均衡"=w3161:dbl)
                    n1265 = call "输入分辨率计算-EV05.vi"("1字节?"=FALSE, "数值"=w3161, "偏移量"=0.0, "分辨率"=0.001) -> ("低字节"=w3163:dbl, "高字节1"=w3165:dbl)  [unwired: 1 in, 5 out]
                  }
                  frame Enabled {
                    w3168 = 255 ("高字节1")
                  }
                }
                n1266 = Build Array(w3160, w3158) -> (w3159:i32[])
              }
              frame 6 {
                # "整组电压不均衡"
                n1267 = disable-structure shown="启用" {
                  disable-tunnel: [w3177 w3180] -> w3172
                  disable-tunnel: [w3175 w3180] -> w3170
                  disable-tunnel: w3169 -> [w3174 _]
                  frame Disabled {
                    n1268 = Unbundle By Name(w3174) -> ("整组电压不均衡"=w3173:dbl)
                    n1269 = call "输入分辨率计算-EV05.vi"("1字节?"=FALSE, "数值"=w3173, "偏移量"=0.0, "分辨率"=0.001) -> ("低字节"=w3175:dbl, "高字节1"=w3177:dbl)  [unwired: 1 in, 5 out]
                  }
                  frame Enabled {
                    w3180 = 255 ("高字节1")
                  }
                }
                n1270 = Build Array(w3172, w3170) -> (w3171:i32[])
              }
              frame 7 {
                # "单体电压过高"
                n1271 = disable-structure shown="启用" {
                  disable-tunnel: [w3189 w3192] -> w3184
                  disable-tunnel: [w3187 w3192] -> w3182
                  disable-tunnel: w3181 -> [w3186 _]
                  frame Disabled {
                    n1272 = Unbundle By Name(w3186) -> ("单体电压过高"=w3185:dbl)
                    n1273 = call "输入分辨率计算-EV05.vi"("1字节?"=FALSE, "数值"=w3185, "偏移量"=0.0, "分辨率"=0.001) -> ("低字节"=w3187:dbl, "高字节1"=w3189:dbl)  [unwired: 1 in, 5 out]
                  }
                  frame Enabled {
                    w3192 = 255 ("高字节1")
                  }
                }
                n1274 = Build Array(w3184, w3182) -> (w3183:i32[])
              }
              frame 8 {
                # "单体电压过低"
                n1275 = disable-structure shown="启用" {
                  disable-tunnel: [w3201 w3204] -> w3196
                  disable-tunnel: [w3199 w3204] -> w3194
                  disable-tunnel: w3193 -> [w3198 _]
                  frame Disabled {
                    n1276 = Unbundle By Name(w3198) -> ("单体电压过低"=w3197:dbl)
                    n1277 = call "输入分辨率计算-EV05.vi"("1字节?"=FALSE, "数值"=w3197, "偏移量"=0.0, "分辨率"=0.001) -> ("低字节"=w3199:dbl, "高字节1"=w3201:dbl)  [unwired: 1 in, 5 out]
                  }
                  frame Enabled {
                    w3204 = 255 ("高字节1")
                  }
                }
                n1278 = Build Array(w3196, w3194) -> (w3195:i32[])
              }
              frame 9 {
                # "充电电流过高"
                n1279 = disable-structure shown="启用" {
                  disable-tunnel: [w3213 w3216] -> w3208
                  disable-tunnel: [w3211 w3216] -> w3206
                  disable-tunnel: w3205 -> [w3210 _]
                  frame Disabled {
                    n1280 = Unbundle By Name(w3210) -> ("充电电流过高"=w3209:dbl)
                    n1281 = call "输入分辨率计算-EV05.vi"("1字节?"=FALSE, "数值"=w3209, "偏移量"=-3000.0, "分辨率"=0.1) -> ("低字节"=w3211:dbl, "高字节1"=w3213:dbl)  [unwired: 1 in, 5 out]
                  }
                  frame Enabled {
                    w3216 = 255 ("高字节1")
                  }
                }
                n1282 = Build Array(w3208, w3206) -> (w3207:i32[])
              }
              frame 10 {
                # "放电电流过高"
                n1283 = disable-structure shown="启用" {
                  disable-tunnel: [w3225 w3228] -> w3220
                  disable-tunnel: [w3223 w3228] -> w3218
                  disable-tunnel: w3217 -> [w3222 _]
                  frame Disabled {
                    n1284 = Unbundle By Name(w3222) -> ("放电电流过高"=w3221:dbl)
                    n1285 = call "输入分辨率计算-EV05.vi"("1字节?"=FALSE, "数值"=w3221, "偏移量"=-3000.0, "分辨率"=0.1) -> ("低字节"=w3223:dbl, "高字节1"=w3225:dbl)  [unwired: 1 in, 5 out]
                  }
                  frame Enabled {
                    w3228 = 255 ("高字节1")
                  }
                }
                n1286 = Build Array(w3220, w3218) -> (w3219:i32[])
              }
              frame 11 {
                # "单组温度不均衡"
                n1287 = disable-structure shown="启用" {
                  disable-tunnel: [w3235 255 ("高字节1")] -> w3231
                  disable-tunnel: w3229 -> [w3233 _]
                  frame Disabled {
                    n1288 = Unbundle By Name(w3233) -> ("单组温度不均衡"=w3232:dbl)
                    n1289 = call "输入分辨率计算-EV05.vi"("1字节?"=TRUE, "数值"=w3232, "偏移量"=0.0, "分辨率"=1.0) -> ("高字节1"=w3235:dbl)  [unwired: 1 in, 6 out]
                  }
                  frame Enabled {
                  }
                }
                n1290 = Build Array(w3231) -> (w3230:i32[])
              }
              frame 12 {
                # "SOC过高"
                n1291 = Unbundle By Name(w3243) -> ("SOC过高"=w3242:dbl)
                n1292 = call "输入分辨率计算-EV05.vi"("1字节?"=FALSE, "数值"=w3242, "偏移量"=0.0, "分辨率"=0.1) -> ("低字节"=w3244:dbl, "高字节1"=w3245:dbl)  [unwired: 1 in, 5 out]
                n1293 = call "二进制解析-8.6.vi"("索引"=4, "数值"=w3245) -> ("低位子数组"=w3248:i32[])  [unwired: 3 out]
                n1294 = call "二进制解析-8.6.vi"("索引"=4, "数值"=w3244) -> ("低位子数组"=w3240:i32[], "高位子数组"=w3247:i32[])  [unwired: 2 out]
                n1295 = Insert Into Array(array=w3248, new element=w3247) -> (w3246:i32[])  [unwired: 1 in]
                n1296 = call "数值二进制转十进制-8.6.vi"("子数组"=w3246) -> ("十进制数值"=w3241:i32)  [unwired: 4 out]
                n1297 = disable-structure shown="启用" {
                  disable-tunnel: w3241 -> [w3256 _]
                  disable-tunnel: [w3256 255 ("高字节1")] -> w3239
                  disable-tunnel: [w3255 i32[] [] ("低位子数组 21")] -> _
                  disable-tunnel: w3240 -> [w3255 _]
                  frame Disabled {
                  }
                  frame Enabled {
                  }
                }
                n1298 = Build Array(w3239, w3239) -> (w3252:i32[])
              }
              frame 13 {
                # "SOC过低"
                n1299 = Unbundle By Name(w3265) -> ("SOC过低"=w3264:dbl)
                n1300 = call "输入分辨率计算-EV05.vi"("1字节?"=FALSE, "数值"=w3264, "偏移量"=0.0, "分辨率"=0.1) -> ("低字节"=w3262:dbl, "高字节1"=w3263:dbl)  [unwired: 1 in, 5 out]
                n1301 = call "二进制解析-8.6.vi"("索引"=4, "数值"=w3263) -> ("低位子数组"=w3260:i32[])  [unwired: 3 out]
                n1302 = disable-structure shown="启用" {
                  disable-tunnel: w3262 -> [w3272 _]
                  disable-tunnel: [w3272 255 ("高字节1")] -> w3261
                  disable-tunnel: w3260 -> [w3271 _]
                  disable-tunnel: [_ 255 ("高字节1")] -> w3259
                  frame Disabled {
                    (unwired) i32[] [] ("低位子数组 4")
                  }
                  frame Enabled {
                  }
                }
                n1303 = Build Array(w3259, w3261) -> (w3268:i32[])
              }
              frame 14 {
                # "内阻过大"
                n1304 = disable-structure shown="启用" {
                  disable-tunnel: w3277 -> [w3282 _]
                  disable-tunnel: [w3278 255 ("高字节1")] -> w3275
                  frame Disabled {
                    n1305 = Unbundle By Name(w3282) -> ("内阻过大"=w3281:dbl)
                    n1306 = call "输入分辨率计算-EV05.vi"("1字节?"=TRUE, "数值"=w3281, "分辨率"=0.1) -> ("高字节1"=w3278:dbl)  [unwired: 2 in, 6 out]
                  }
                  frame Enabled {
                  }
                }
                n1307 = Build Array(w3275) -> (w3276:i32[])
              }
              frame 15 {
                # "极柱温度过高"
                n1308 = disable-structure shown="启用" {
                  disable-tunnel: w3286 -> [w3292 _]
                  disable-tunnel: [w3288 255 ("高字节1")] -> w3284
                  frame Disabled {
                    n1309 = Unbundle By Name(w3292) -> ("极柱温度过高"=w3291:dbl)
                    n1310 = call "输入分辨率计算-EV05.vi"("1字节?"=TRUE, "数值"=w3291, "偏移量"=-40.0, "分辨率"=1.0) -> ("高字节1"=w3288:dbl)  [unwired: 1 in, 6 out]
                  }
                  frame Enabled {
                  }
                }
                n1311 = Build Array(w3284) -> (w3285:i32[])
              }
              frame 16 {
                # "SOH过低"
                n1312 = disable-structure shown="启用" {
                  disable-tunnel: [w3309 w3317] -> w3296
                  disable-tunnel: w3295 -> [w3306 _]
